vi "henghui_PLD_3605_control1.vi"() -> ()   [LabVIEW 2019]
uses:
  <vilib>/Instr/_visa.llb/VISA Configure Serial Port (Instr).vi
panel:
  out "x-y":u32
  in  "stop":bool
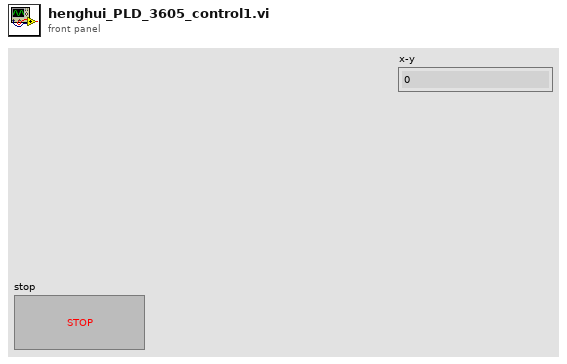
[diagram p1: front panel]
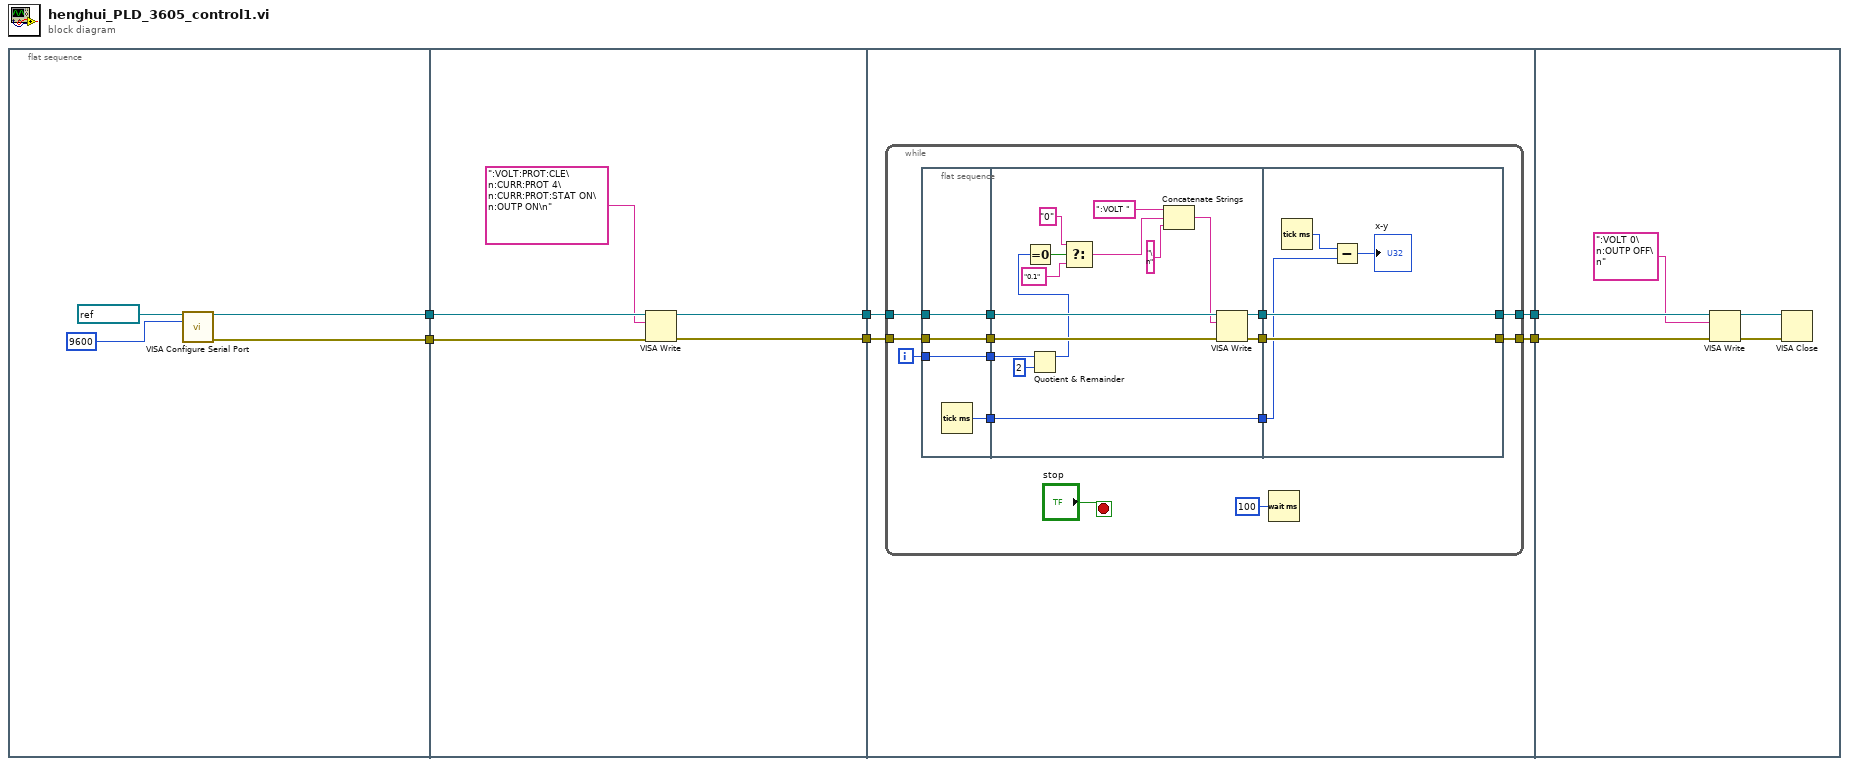
[diagram p0: block diagram]
diagram:
  n1 = flat-sequence {
    tunnel: [w8] -> w6
    tunnel: [w7] -> w5
    tunnel: w6 -> [w15]
    tunnel: w5 -> [w14]
    tunnel: [w12] -> w4
    tunnel: [w11] -> w3
    tunnel: w4 -> [w19]
    tunnel: w3 -> [w18]
    tunnel: [w17] -> w2
    tunnel: [w16] -> w1
    tunnel: w2 -> [w62]
    tunnel: w1 -> [w61]
    frame #0 {
      n2 = call-poly "VISA Configure Serial Port"("VISA resource name"=refnum<visa-resource-name> "COM8", "baud rate (9600)"=u32 9600) -> ("VISA resource name out"=w8:refnum<visa-resource-name>, "error out"=w7:errorcluster)  [unwired: 12 in]
    }
    frame #1 {
      n3 = VISA Write(VISA resource name=w15, write buffer=":VOLT:PROT:CLE\n:CURR:PROT 4\n:CURR:PROT:STAT ON\n:OUTP ON\n", error in (no error)=w14) -> (VISA resource name out=w12:refnum<visa-resource-name>, error out=w11:errorcluster)  [unwired: 1 out]
    }
    frame #2 {
      n4 = while {
        tunnel: [w29] -> w17
        tunnel: w19 -> [w31]
        tunnel: w18 -> [w30]
        tunnel: [w28] -> w16
        i -> [w22]
        stop <- "stop" stop-if-true
        n5 = flat-sequence {
          tunnel: w30 -> [w36]
          tunnel: w31 -> [w37]
          tunnel: [w37] -> w27
          tunnel: [w36] -> w26
          tunnel: [w35] -> w23
          tunnel: w22 -> [w35]
          tunnel: [w34] -> w21
          tunnel: w27 -> [w52]
          tunnel: w26 -> [w51]
          tunnel: [w50] -> w25
          tunnel: [w49] -> w24
          tunnel: w23 -> [w45]
          tunnel: w21 -> [w38]
          tunnel: [w38] -> w20
          tunnel: [w56] -> w28
          tunnel: [w57] -> w29
          tunnel: w25 -> [w57]
          tunnel: w24 -> [w56]
          tunnel: w20 -> [w54]
          frame #0 {
            n6 = Tick Count (ms)() -> (millisecond timer value=w34:u32)
          }
          frame #1 {
            n7 = Quotient & Remainder(x=w45, y=2) -> (x-y*floor(x/y)=w42:i32)  [unwired: 1 out]
            n8 = Equal To 0?(x=w42) -> (x = 0?=w43:bool)
            n9 = Select(t="0" ("write buffer"), s=w43, f="0.1" ("write buffer")) -> (s? t:f=w39:string)
            n10 = Concatenate Strings(":VOLT " ("write buffer"), w39, "\n" ("string")) -> (w46:string)
            n11 = VISA Write(VISA resource name=w52, write buffer=w46, error in (no error)=w51) -> (VISA resource name out=w50:refnum<visa-resource-name>, error out=w49:errorcluster)  [unwired: 1 out]
          }
          frame #2 {
            n12 = Tick Count (ms)() -> (millisecond timer value=w55:u32)
            n13 = Subtract(x=w55, y=w54) -> (x-y=→"x-y":u32)
          }
        }
        n14 = Wait (ms)(milliseconds to wait=u32 100) -> ()  [unwired: 1 out]
      }
    }
    frame #3 {
      n15 = VISA Write(VISA resource name=w62, write buffer=":VOLT 0\n:OUTP OFF\n", error in (no error)=w61) -> (VISA resource name out=w59:refnum<visa-resource-name>, error out=w58:errorcluster)  [unwired: 1 out]
      n16 = VISA Close(VISA resource name=w59, error in (no error)=w58) -> ()  [unwired: 1 out]
    }
  }
